vi "Create Function String (Delta).vi"(8 "error in (no error)":errorcluster, 9 "Wiring Unit (7: Sigma A)":i32(ring)=7 items=["Sigma A"=7, "Sigma B"=8, "Sigma C"=9], 10 "Function (0: Delta U1)":i32(ring) items=["Delta U1", "Delta U2", "Delta U3", "Delta U Sigma", "Delta I", "Delta P1", "Delta P2", "Delta P3", "Delta P Sigma"], 11 "VISA resource name":refnum<visa-resource-name>) -> (0 "error out":errorcluster, 2 "Function String":string, 3 "VISA resource name out":refnum<visa-resource-name>)   [LabVIEW 2021, in "Yokogawa WT1800 Series.lvlib"]
doc: "Create a delta function string.\n\n<b>Note:</b>\nThis setting valid on models with the delta computation (/DT) option."
uses:
  <instrlib>/Yokogawa WT1800 Series/Yokogawa WT1800 Series.lvlib
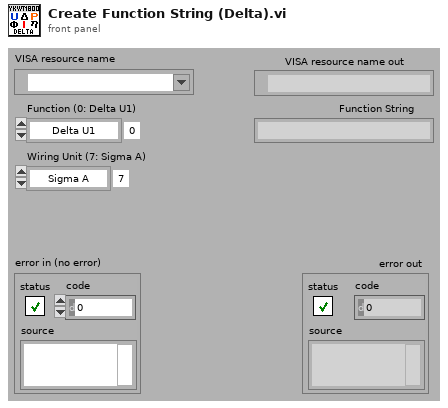
[diagram p1: front panel]
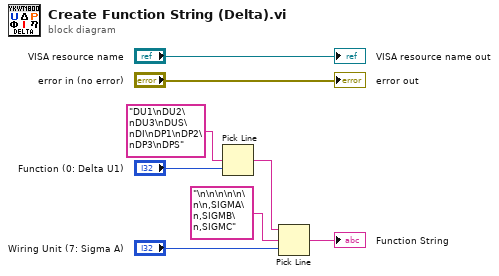
[diagram p0: block diagram]
diagram:
  n1 = Pick Line ("ライン選択")(multi-line string="DU1\nDU2\nDU3\nDUS\nDI\nDP1\nDP2\nDP3\nDPS" ("複数行文字列"), line index="Function (0: Delta U1)") -> (output string=w4:string)  [unwired: 1 in]
  n2 = Pick Line ("ライン選択")(string ("")=w4, multi-line string="\n\n\n\n\n\n\n,SIGMA\n,SIGMB\n,SIGMC" ("複数行文字列"), line index="Wiring Unit (7: Sigma A)") -> (output string=→"Function String":string)
  "VISA resource name out" <- "VISA resource name"
  "error out" <- "error in (no error)"
